vi "Theta 1.vi"(9 "AB":dbl[](array[numeric]), 10 "theta_2":dbl, 11 "6R Type 3 Serial Arm Class in":refnum<class "NI_Robotics_6R Type 3 Serial Arm Class.lvclass">) -> (1 "valid?":bool, 2 "theta_1":dbl, 3 "6R Type 3 Serial Arm Class out":refnum<class "NI_Robotics_6R Type 3 Serial Arm Class.lvclass">)   [LabVIEW 2017, in "NI_Robotics_6R Type 3 Serial Arm Class.lvclass"]
uses:
  <vilib>/robotics/Kinematics/Analytical/6R/Type 3/NI_Robotics_6R Type 3 Serial Arm Class.lvclass
  c:/Program Files (x86)/National Instruments/LabVIEW 2017/vi.lib/robotics/Kinematics/Analytical/Generic/NI_Robotics_Analytical Serial Arm Class.lvclass
  <vilib>/Analysis/7linalg.llb/Solve Linear Equations (single right hand).vi
  <vilib>/Analysis/baseanly.llb/Solve Linear Equations By Cholesky.vi
  <vilib>/Analysis/baseanly.llb/Real Matrix to Compact Array.vi
  <vilib>/Analysis/baseanly.llb/Real Compact Tri-Matrix Linear Eqs.vi
  <vilib>/Analysis/7linalg.llb/Solve Linear Eqs (General).vi
  <vilib>/Analysis/7linalg.llb/Solve Linear Eqs (Gen, single right hand).vi
  <vilib>/Analysis/NI_AALPro.lvlib
  <vilib>/robotics/Kinematics/Analytical/Generic/NI_Robotics_Analytical Serial Arm Class.lvclass
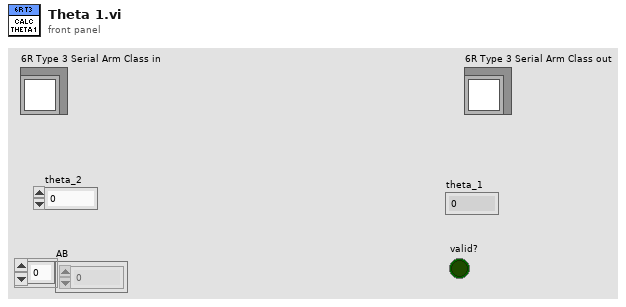
[diagram p1: front panel]
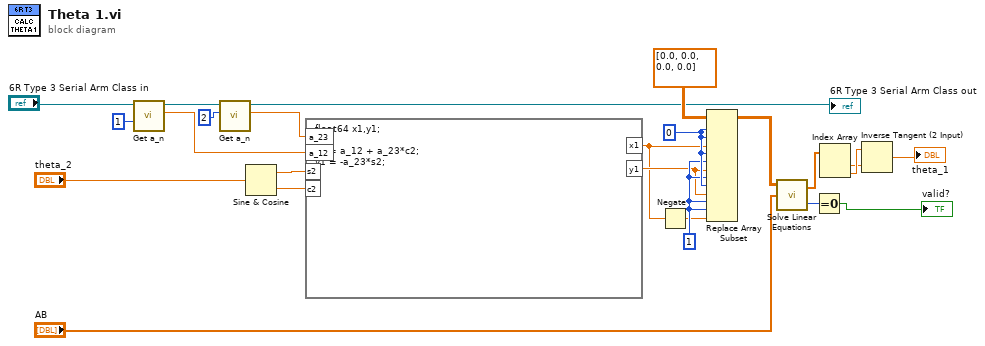
[diagram p0: block diagram]
diagram:
  w14 = 1 ("disabled index (col)")
  w15 = 0 ("index (row)")
  n1 = call <vilib>:"Get a_n.vi"("n"=1, "Analytical Serial Arm Class in"="6R Type 3 Serial Arm Class in") -> ("a_n"=w19:dbl, "Analytical Serial Arm Class out"=w22:refnum<class "NI_Robotics_6R Type 3 Serial Arm Class.lvclass">)  [unwired: 8 in]
  n2 = call <vilib>:"Get a_n.vi"("n"=2, "Analytical Serial Arm Class in"=w22) -> ("a_n"=w20:dbl, "Analytical Serial Arm Class out"=→"6R Type 3 Serial Arm Class out":refnum<class "NI_Robotics_6R Type 3 Serial Arm Class.lvclass">)  [unwired: 8 in]
  n3 = Sine & Cosine(0:"theta_2") -> (1:w18:dbl, 2:w17:dbl)
  n4 = formula code="float64 x1,y1;\n\nx1 = a_12 + a_23*c2;\ny1 = -a_23*s2;"("a_23"=w20, "a_12"=w19, "s2"=w18, "c2"=w17) -> ("x1"=w10:dbl, "y1"=w12:dbl)
  n5 = Negate(x=w10) -> (-x=w9:dbl)
  n6 = Replace Array Subset(array=dbl[][] [[0.0, 0.0], [0.0, 0.0]], new element #1=w10, index (row) #1=w15, index (col) #1=w15, new element #2=w12, index (row) #2=w15, index (col) #2=w14, new element #3=w12, index (row) #3=w14, index (col) #3=w15, new element #4=w9, index (row) #4=w14, index (col) #4=w14) -> (w4:dbl[][])
  n7 = call-poly <vilib>:"Solve Linear Equations.vi"("Known Vector"="AB", "Input Matrix"=w4) -> ("error"=w8:i32, "Solution Vector"=w5:dbl[])  [unwired: 1 in]
  n8 = Equal To 0?(x=w8) -> (x = 0?=→"valid?":bool)
  n9 = Index Array(array=w5) -> (element #1=w6:dbl, element #2=w7:dbl)  [unwired: 2 in]
  n10 = Inverse Tangent (2 Input)(1:w6, 2:w7) -> (0:→"theta_1":dbl)
